vi "IsCapturing.vi"(8 "error in (no error)":errorcluster, 11 "Camera in":refnum<class "Camera.lvclass">) -> (0 "error out":errorcluster, 2 "isBusy?":bool, 3 "Camera out":refnum<class "Camera.lvclass">)   [LabVIEW 2020]
uses:
  Camera.lvclass
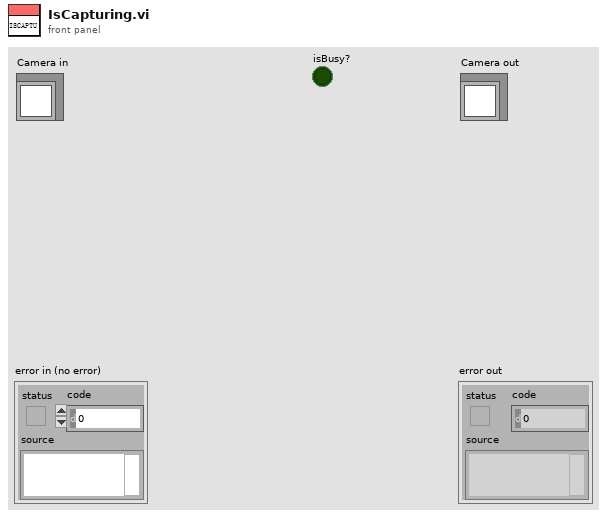
[diagram p1: front panel]
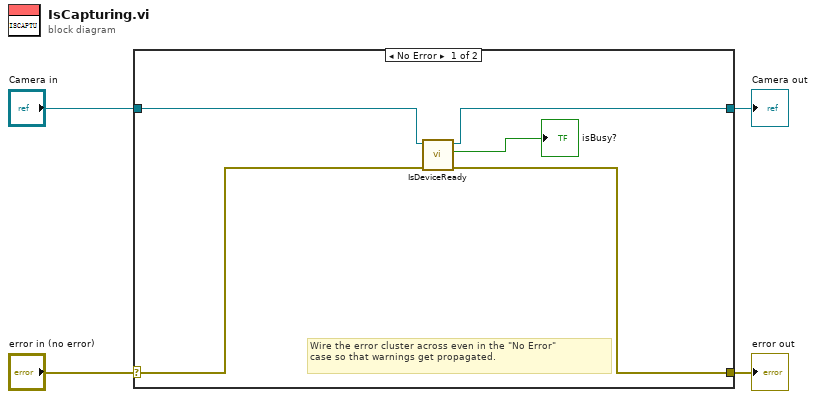
[diagram p0: block diagram]
diagram:
  n1 = case shown="No Error" "error in (no error)" {
    selector: "error in (no error)" -> [w6 w11]
    tunnel: [w7 w11] -> w3
    tunnel: [w8 w10] -> w1
    tunnel: "Camera in" -> [w9 w10]
    frame No Error {
      # "Wire the error cluster across even in the \"No Error\"\ncase so that warnings get propagated."
      n2 = call-dynamic "IsDeviceReady.vi"("error in (no error)"=w6, "Device in"=w9) -> ("error out"=w7:errorcluster, "Ready?"=→"isBusy?":bool, "Device out"=w8:refnum<class "Camera.lvclass">)  [unwired: 7 in]
    }
    frame Error {
    }
  }
  "error out" <- w3
  "Camera out" <- w1
